vi "FTW-Container-Load-JSON.vi"(0 "Container":refnum<class "FTW-Container.lvclass">, 5 "JSON to Load":string, 11 "error in":errorcluster) -> (4 "Container out":refnum<class "FTW-Container.lvclass">, 6 "Serialized Node":string, 15 "error out":errorcluster)   [LabVIEW 2013, in "FTW-Container.lvclass"]
uses:
  FTW-Container.lvclass
  FTW-Container.lvclass/FTW-Container.ctl
panel:
  # "Inputs"
  # "Outputs"
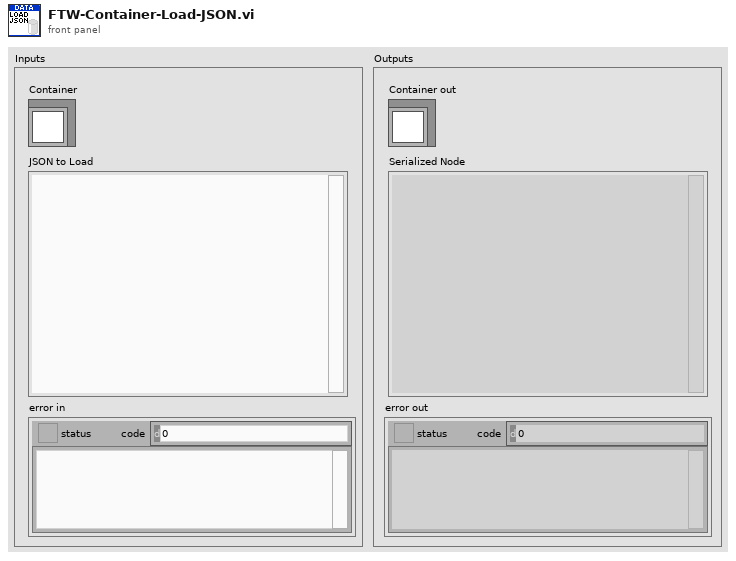
[diagram p1: front panel]
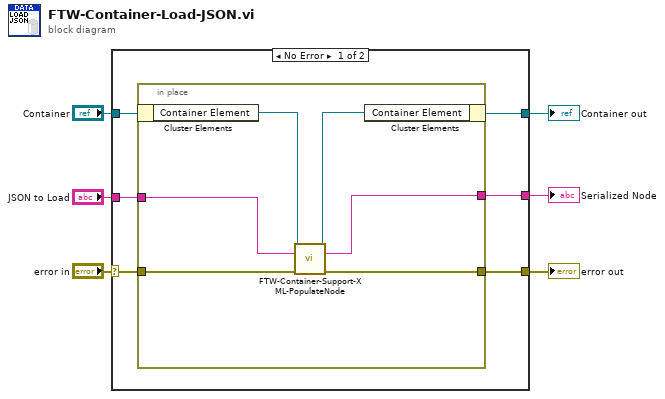
[diagram p0: block diagram]
diagram:
  n1 = case shown="No Error" "error in" {
    selector: "error in" -> [w12 w20]
    tunnel: [w11 w20] -> w6
    tunnel: "Container" -> [w10 w19]
    tunnel: [w9 w19] -> w3
    tunnel: "JSON to Load" -> [w8 _]
    tunnel: [w7 _] -> w1
    frame No Error {
      n2 = in-place {
        in-place-border: w12 -> [w16]
        in-place-border: [w15] -> w11
        in-place-border: w8 -> [w14]
        in-place-border: [w13] -> w7
        n3 = in-place-cluster #1(w10) -> ("Container Element"=w18:refnum<k20>)
        n4 = call "FTW-Container-Support-XML-PopulateNode.vi"("Element Node"=w18, "JSON"=w14, "error in"=w16) -> ("Element Node out"=w17:refnum<k20>, "Serialized Node"=w13:string, "error out"=w15:errorcluster)  [unwired: 10 in]
        n5 = in-place-cluster #1("Container Element"=w17) -> (w9:refnum<class "FTW-Container.lvclass">)
      }
    }
    frame Error {
    }
  }
  "error out" <- w6
  "Container out" <- w3
  "Serialized Node" <- w1
